vi "ExecuteCommand.vi"(10 "Params":string[][](array[string]), 11 "Command":string) -> ()   [LabVIEW 2017]
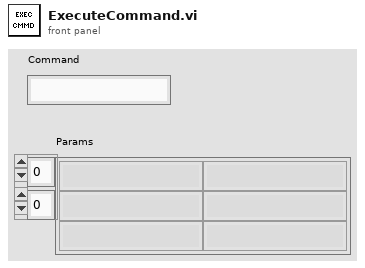
[diagram p1: front panel]
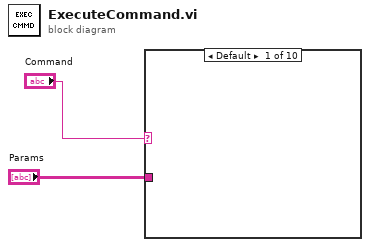
[diagram p0: block diagram]
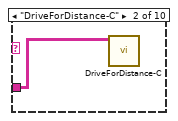
[diagram p2: hidden frame]
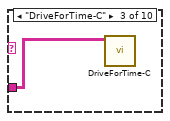
[diagram p3: hidden frame]
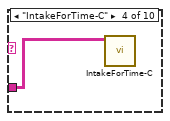
[diagram p4: hidden frame]
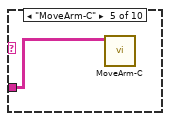
[diagram p5: hidden frame]
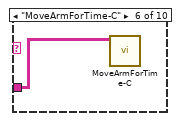
[diagram p6: hidden frame]
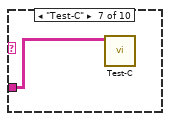
[diagram p7: hidden frame]
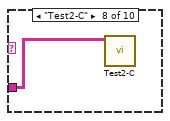
[diagram p8: hidden frame]
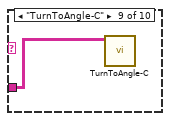
[diagram p9: hidden frame]
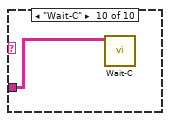
[diagram p10: hidden frame]
diagram:
  n1 = case shown="Default" "Command" {
    tunnel: "Params" -> [_ w3 w4 w5 w6 w7 w8 w9 w10 w11]
    frame Default {
    }
    frame "DriveForDistance-C" {
      n2 = call "DriveForDistance-C.vi"("Params"=w3) -> ()  [unwired: 11 in]
    }
    frame "DriveForTime-C" {
      n3 = call "DriveForTime-C.vi"("Params"=w4) -> ()  [unwired: 11 in]
    }
    frame "IntakeForTime-C" {
      n4 = call "IntakeForTime-C.vi"("Params"=w5) -> ()  [unwired: 11 in]
    }
    frame "MoveArm-C" {
      n5 = call "MoveArm-C.vi"("Params"=w6) -> ()  [unwired: 11 in]
    }
    frame "MoveArmForTime-C" {
      n6 = call "MoveArmForTime-C.vi"("Params"=w7) -> ()  [unwired: 11 in]
    }
    frame "Test-C" {
      n7 = call "Test-C.vi"("Params"=w8) -> ()  [unwired: 11 in]
    }
    frame "Test2-C" {
      n8 = call "Test2-C.vi"("Params"=w9) -> ()  [unwired: 11 in]
    }
    frame "TurnToAngle-C" {
      n9 = call "TurnToAngle-C.vi"("Params"=w10) -> ()  [unwired: 11 in]
    }
    frame "Wait-C" {
      n10 = call "Wait-C.vi"("Params"=w11) -> ()  [unwired: 11 in]
    }
  }
